vi "CheckRealCollide.vi"(8 "IntensityArray_IN":u8[][](array[numeric]), 11 "ShotPosition":T1) -> (3 "RealCollide?":bool)   [LabVIEW 2022 SP3]
panel:
  out "subarray":dbl[][](array[numeric])
  in  "length 2":i32
  in  "index 2":i32
  in  "length":i32
  in  "index":i32
  in  "array":dbl[][](array[numeric])
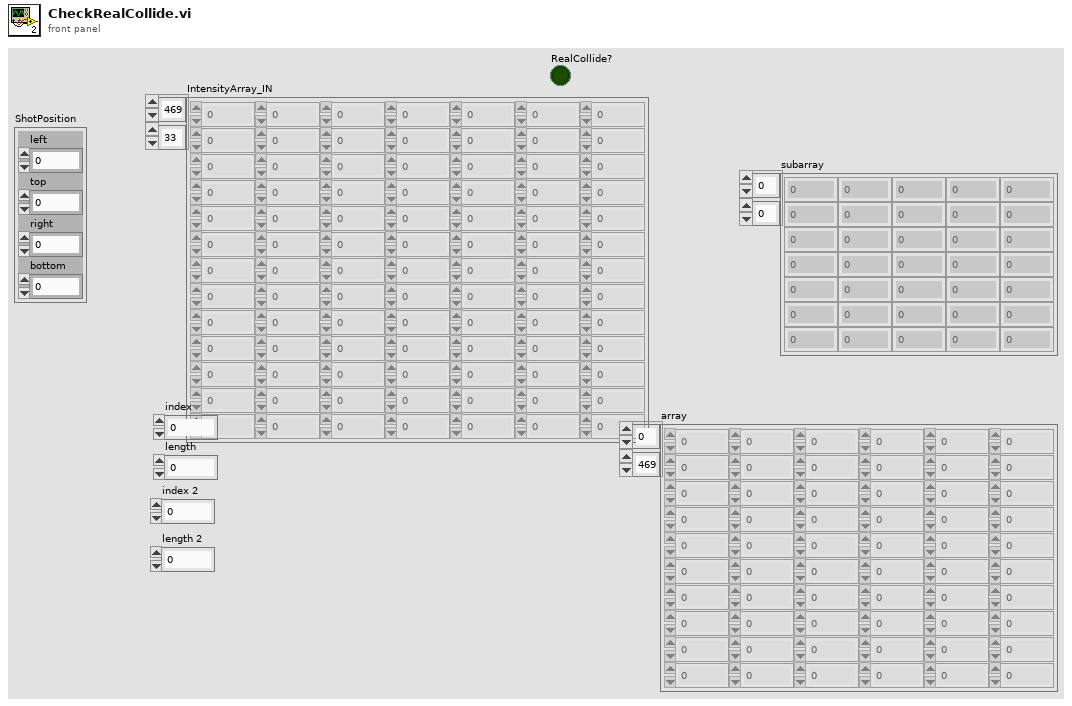
[diagram p1: front panel]
types:
  T1 = cluster{"left":i16, "top":i16, "right":i16, "bottom":i16}
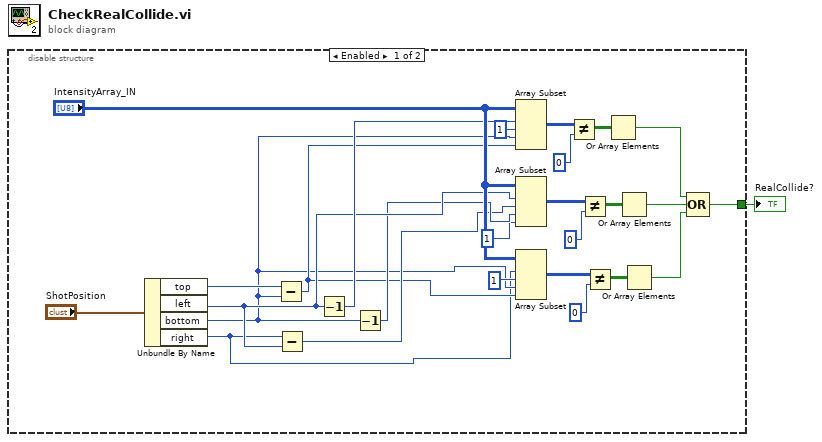
[diagram p0: block diagram]
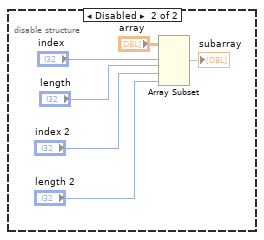
[diagram p2: hidden frame]
diagram:
  n1 = disable-structure shown="Enabled" {
    disable-tunnel: [w12 _] -> w1
    frame Enabled {
      n2 = Unbundle By Name("ShotPosition") -> ("top"=w25:i16, "left"=w9:i16, "bottom"=w3:i16, "right"=w2:i16)
      n3 = Subtract(x=w25, y=w3) -> (x-y=w4:i16)
      n4 = Subtract(x=w2, y=w9) -> (x-y=w6:i16)
      n5 = Decrement(x=w9) -> (x-1=w11:i16)
      n6 = Decrement(x=w3) -> (x-1=w8:i16)
      n7 = Array Subset(array="IntensityArray_IN", index (row)=w11, length (row)=1 ("length"), index (col)=w3, length (col)=w4) -> (w24:u8[][])
      n8 = Array Subset(array="IntensityArray_IN", index (row)=w9, length (row)=w6, index (col)=w8, length (col)=1 ("length")) -> (w19:u8[][])
      n9 = Array Subset(array="IntensityArray_IN", index (row)=w2, length (row)=1 ("length"), index (col)=w3, length (col)=w4) -> (w16:u8[][])
      n10 = Not Equal?(x=w24, y=u8 0 ("element")) -> (x != y?=w22:bool[][])
      n11 = Not Equal?(x=w19, y=u8 0 ("element")) -> (x != y?=w21:bool[][])
      n12 = Not Equal?(x=w16, y=u8 0 ("element")) -> (x != y?=w17:bool[][])
      n13 = Or Array Elements(Boolean array=w22) -> (logical OR=w15:bool)
      n14 = Or Array Elements(Boolean array=w21) -> (logical OR=w14:bool)
      n15 = Or Array Elements(Boolean array=w17) -> (logical OR=w13:bool)
      n16 = Compound Arithmetic op=OR(w15, w14, w13) -> (w12:bool)
    }
    frame Disabled {
      n17 = Array Subset(array="array", index (row)="index", length (row)="length", index (col)="index 2", length (col)="length 2") -> (→"subarray":dbl[][])
    }
  }
  "RealCollide?" <- w1
